vi "CheckImage.vi"(7 "Color System":u16(ring)=2 items=["RGB", "HSL", "HSV", "HSI"], 10 "Image":T2, 11 "Color Components":T3={"Hue"={110.0, 142.0}, "Sat"={138.0, 255.0}, "Val"={139.0, 198.0}} {"Val" scale=0.0..255.0; "Sat" scale=0.0..255.0; "Hue" scale=0.0..255.0 scale format="%#_3g"}) -> (0 "Distance (ft)":dbl, 1 "Scores.State":T1, 2 "Image out":T2)   [LabVIEW 2013]
uses:
  <vilib>/vision/Image Controls.llb/IMAQ Image.ctl
  Example_Code/2014 Target Detection/TargetType.ctl
panel:
  in  "Camera Type":enum16{"206", "1011", "1013"}(ring)=enum."1013"
  in  "Score Cutoff":dbl(slide)=54.248366013071895 scale=0.0..100.0
  in  "Area Size Limit %":dbl=0.06 format="%#_13g"
  out "Mask":T2(plugin-control)
  out "Image":T2(plugin-control)
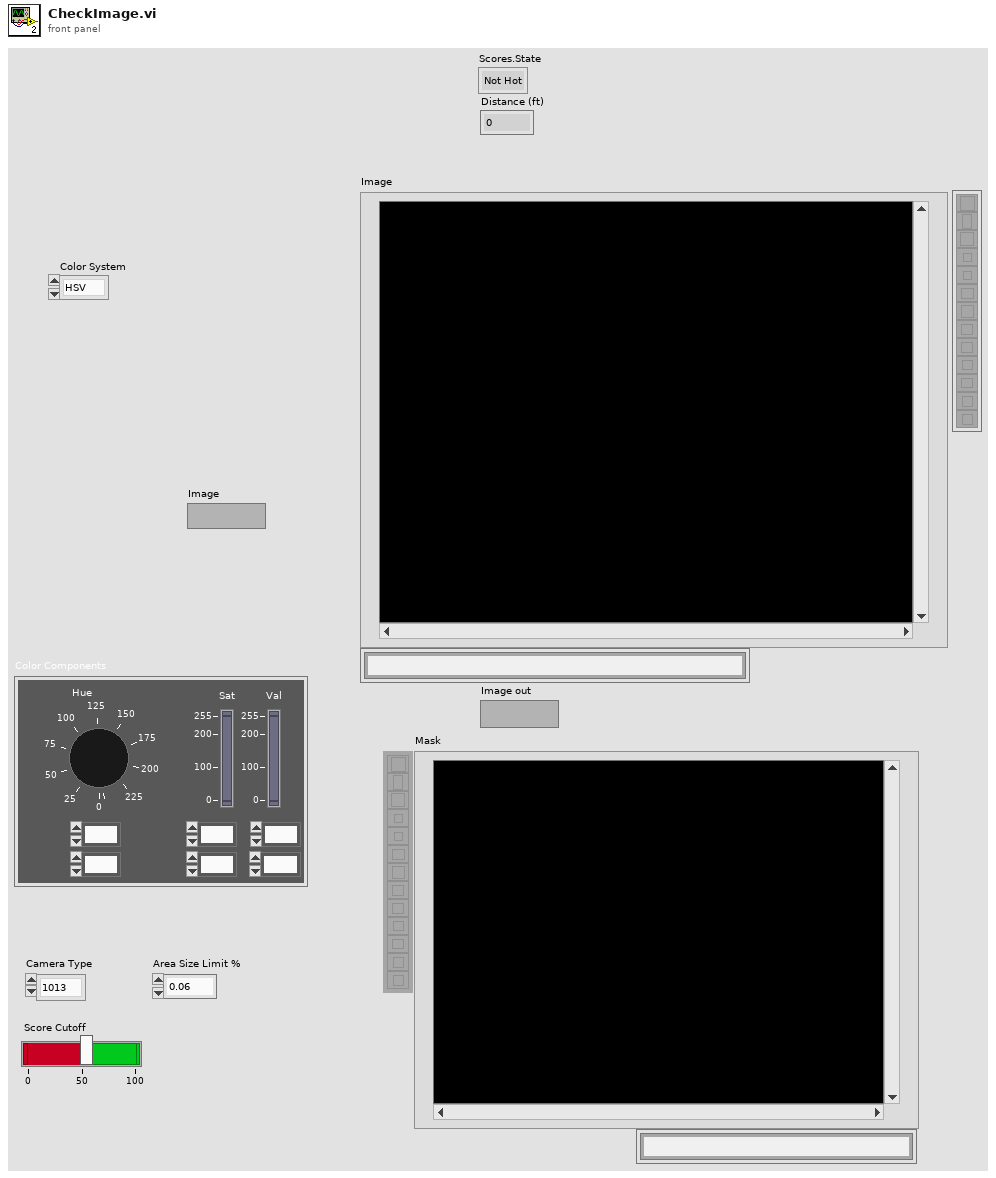
[diagram p1: front panel]
types:
  T1 = typedef "TargetType.ctl" = enum16{"Not Hot", "Hot"}
  T2 = typedef "IMAQ Image.ctl" = refnum<image>
  T3 = cluster{"Hue":cluster{dbl, dbl}, "Sat":cluster{dbl, dbl}, "Val":cluster{dbl, dbl}}
  T4 = cluster{"Horizontal":bool, "Aspect Score":dbl, "Rect Score":dbl, cluster{"Left":dbl, "Top":dbl, "Right":dbl, "Bottom":dbl}, "Equiv H":dbl, "Equiv V":dbl}[]
  T5 = cluster{"Scores":cluster{"Total":dbl, "Left":dbl, "Right":dbl, "Ratio":dbl, "Vertical":dbl, "index":i32, "State":T1}, "Verticals":cluster{"Horizontal?":bool, "Aspect Score":dbl, "Rect Score":dbl, cluster{"Left":dbl, "Top":dbl, "Right":dbl, "Bottom":dbl}, "Equiv H":dbl, "Equiv V":dbl}, "Horizontals":cluster{"Horizontal?":bool, "Aspect Score":dbl, "Rect Score":dbl, cluster{"Left":dbl, "Top":dbl, "Right":dbl, "Bottom":dbl}, "Equiv H":dbl, "Equiv V":dbl}, "Validated":bool}[]
  T6 = cluster{"Scores":cluster{"Total":dbl, "Left":dbl, "Right":dbl, "Ratio":dbl, "Vertical":dbl, "index":i32, "State":T1}, "Verticals":cluster{"Horizontal?":bool, "Aspect Score":dbl, "Rect Score":dbl, cluster{"Left":dbl, "Top":dbl, "Right":dbl, "Bottom":dbl}, "Equiv H":dbl, "Equiv V":dbl}, "Horizontals":cluster{"Horizontal?":bool, "Aspect Score":dbl, "Rect Score":dbl, cluster{"Left":dbl, "Top":dbl, "Right":dbl, "Bottom":dbl}, "Equiv H":dbl, "Equiv V":dbl}, "Distance (ft)":dbl, "Target Center (-1 to 1)":cluster{"X":dbl, "Y":dbl}}[]
  T7 = cluster{"Scores":cluster{"Total":dbl, "Left":dbl, "Right":dbl, "Ratio":dbl, "Vertical":dbl, "index":i32, "State":T1}, "Verticals":cluster{"Horizontal?":bool, "Aspect Score":dbl, "Rect Score":dbl, cluster{"Left":dbl, "Top":dbl, "Right":dbl, "Bottom":dbl}, "Equiv H":dbl, "Equiv V":dbl}, "Horizontals":cluster{"Horizontal?":bool, "Aspect Score":dbl, "Rect Score":dbl, cluster{"Left":dbl, "Top":dbl, "Right":dbl, "Bottom":dbl}, "Equiv H":dbl, "Equiv V":dbl}, "Distance (ft)":dbl, "Target Center (-1 to 1)":cluster{"X":dbl, "Y":dbl}}
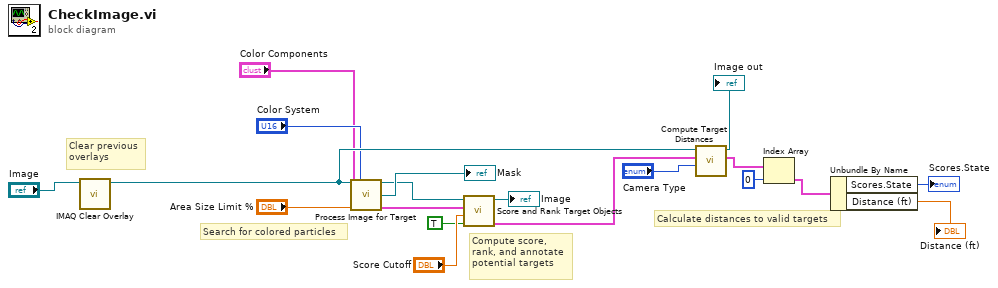
[diagram p0: block diagram]
diagram:
  # "Clear previous\noverlays"
  # "Calculate distances to valid targets"
  # "Search for colored particles"
  # "Compute score,\nrank, and annotate\npotential targets"
  n1 = call "IMAQ Clear Overlay"("Image"="Image") -> ("Image Out"=w11:T2)  [unwired: 9 in, 1 out]
  n2 = call "Process Image for Target.vi"("Src Image"=w11, "Color Mode"="Color System", "Color Components"="Color Components", "Area Cutoff %"="Area Size Limit %") -> ("Src Image Out"=w17:T2, "Threshold"=→"Mask":T2, "Particles"=w14:T4)  [unwired: 9 in]
  n3 = call "Score and Rank Target Objects.vi"("Annotate"=TRUE, "Score Limit"="Score Cutoff", "Particles"=w14, "Image in"=w17) -> ("Target Info"=w13:T5, "Annotated Image"=→"Image":T2)  [unwired: 6 in]
  n4 = call "Compute Target Distances.vi"("Camera Type"="Camera Type", "Target Info"=w13, "Image in"=w11) -> ("Target Info"=w5:T6, "Image out"=→"Image out":T2)  [unwired: 6 in, 1 out]
  n5 = Index Array(array=w5, index=0) -> (element=w3:T7)
  n6 = Unbundle By Name(w3) -> ("Scores.State"=→"Scores.State":T1, "Distance (ft)"=→"Distance (ft)":dbl)
